vi "Fiducical Parameters Finder with joystick.vi"() -> ()   [LabVIEW 2011]
uses:
  Shared Components/Gantry Class/Type Definitions/Init_Modes.ctl
  Shared Components/Gantry Class/Gantry Class.lvclass
  Shared Components/Config Manager Class/Type Definitions/Camera Enum.ctl
  Shared Components/gVision API/gVision/gVision.lvlib
panel:
  out "error out":errorcluster
  in  "Find Fiducial":bool
  out "Preview":T1(plugin-control)
  in  "Stop":bool
  in  "Display Steps":bool
  out "Result":T1(plugin-control)
  out "ficucial coordinates":cluster{"x":dbl, "y":dbl}[](array[cluster])
  in  "Fiducial Parameters":T2
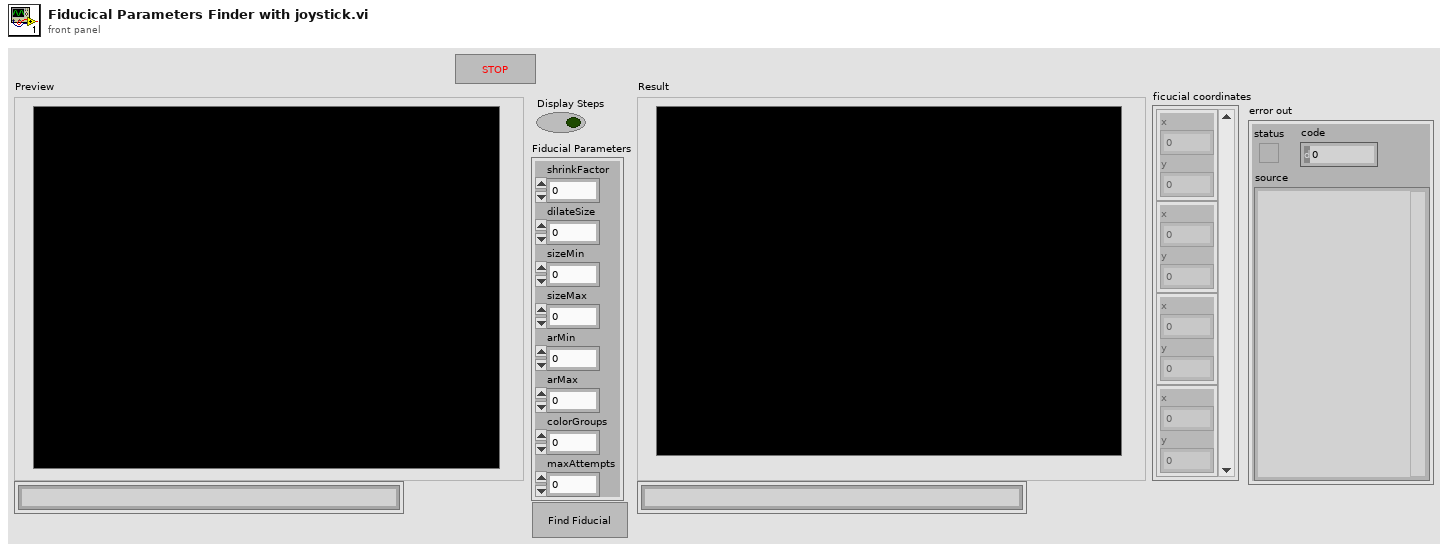
[diagram p1: front panel]
types:
  T1 = typedef "IMAQ Image.ctl" = refnum<image>
  T2 = cluster{"shrinkFactor":sgl, "dilateSize":i32, "sizeMin":sgl, "sizeMax":sgl, "arMin":sgl, "arMax":sgl, "colorGroups":i32, "maxAttempts":i32}
  T3 = typedef "Init_Modes.ctl" = enum16{"Full", "Robot Only", "Dispenser Only", "Cameras Only", "Robot and Cameras", "Robot and Cameras and Dispenser"}
  T4 = cluster{"Left":i32, "Top":i32, "Right":i32, "Bottom":i32}
  T5 = typedef "Camera Enum.ctl" = enum16{"GANTRY HEAD", "NEEDLE CALIBRATION X", "NEEDLE CALIBRATION Y", "STAND CAMERA"}
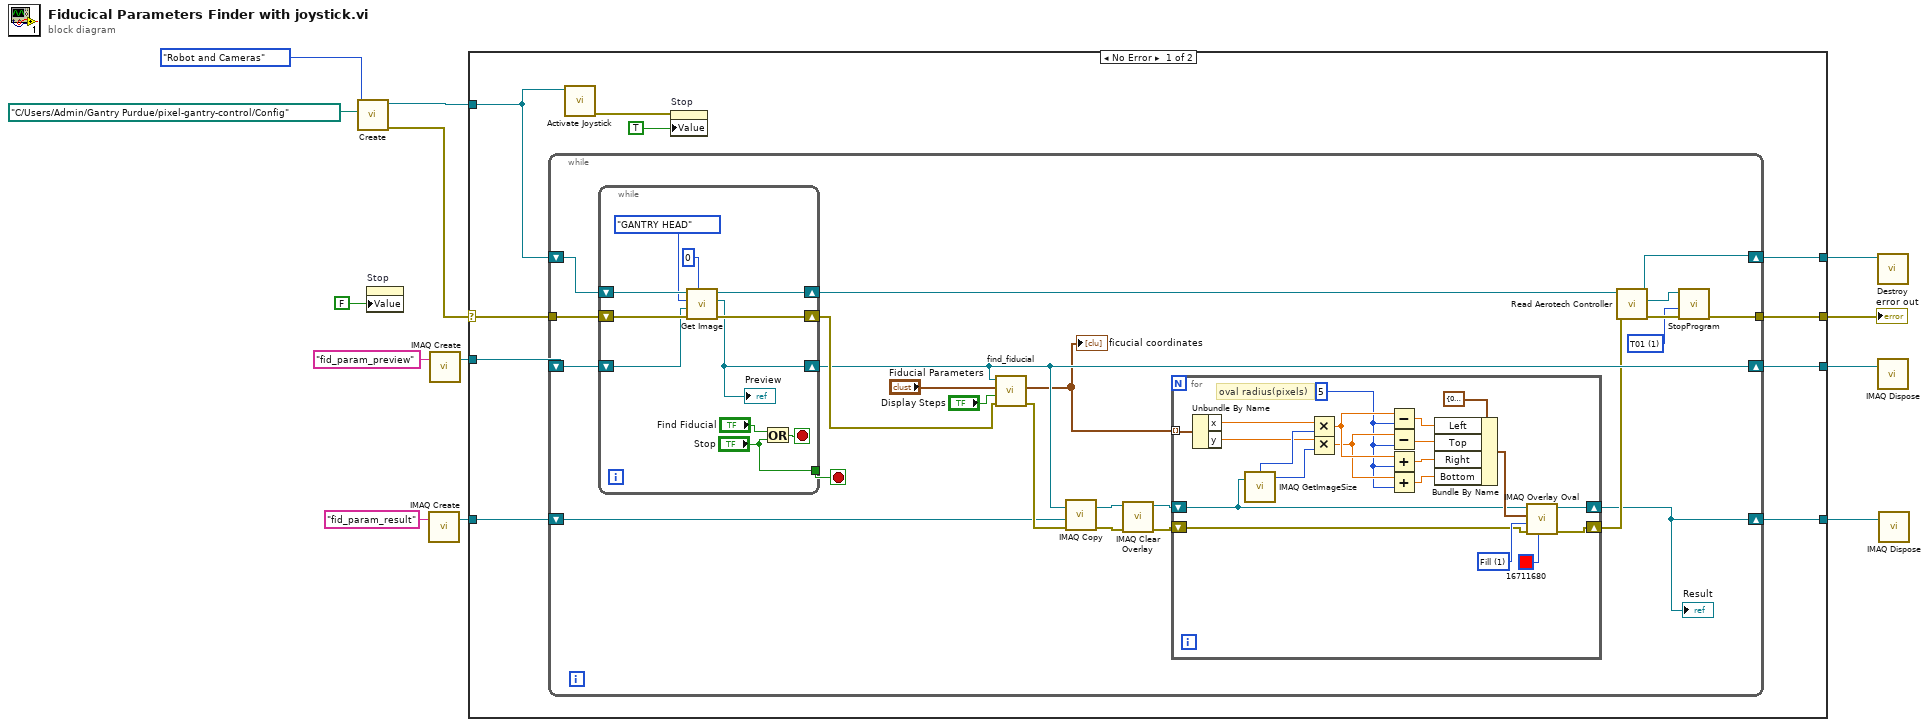
[diagram p0: block diagram]
diagram:
  n1 = call "Create.vi"("Config Folder"=path "C:/Users/Admin/Gantry Purdue/pixel-gantry-control/Config", "Init Mode"=Init_Modes."Robot and Cameras") -> ("error out"=w6:errorcluster, "Gantry out"=w7:refnum<class "Gantry Class.lvclass">)  [unwired: 8 in]
  n2 = property on="Stop" class="Bool (strict)"("Value"=FALSE ("Stop")) -> ()  [unwired: 2 in, 2 out]
  n3 = call "IMAQ Create"("Image Name"="fid_param_result") -> ("New Image"=w9:T1)  [unwired: 4 in, 1 out]
  n4 = call "IMAQ Create"("Image Name"="fid_param_preview") -> ("New Image"=w13:T1)  [unwired: 4 in, 1 out]
  n5 = case shown="No Error" w6 {
    selector: w6 -> [w20 w79]
    tunnel: w13 -> [w23 w81]
    tunnel: [w22 w81] -> w12
    tunnel: w9 -> [w15 w78]
    tunnel: w7 -> [w21 w80]
    tunnel: [w14 w79] -> w3
    tunnel: [w17 w80] -> w8
    tunnel: [w16 w78] -> w1
    frame No Error {
      n6 = while {
        tunnel: w20 -> [w46]
        shift-right: [w40] -> w22
        shift-left: w23 -> [w44]
        shift-right: [w28] -> w17
        shift-left: w21 -> [w45]
        tunnel: [w25] -> w14
        shift-right: [w24] -> w16
        shift-left: w15 -> [w27]
        stop <- w41 stop-if-true
        w31 = 1 items=["TLibrary", "T01", "T02", "T03", "T04", "T05", "T06", "T07", "T08", "T09", "T10", "T11", "T12", "T13", "T14", "T15", "T16", "T17", "T18", "T19", "T20", "T21", "T22", "T23", "T24", "T25", "T26", "T27", "T28", "T29", "T30", "T31"] ("taskId")
        n7 = while {
          shift-right: [w72] -> w40
          shift-left: w44 -> [w75]
          shift-right: [w74] -> w29
          shift-left: w45 -> [w76]
          shift-right: [w73] -> w42
          shift-left: w46 -> [w77]
          tunnel: ["Stop"] -> w41
          stop <- w70 stop-if-true
          n8 = call-dynamic "Get Image.vi"("Delay(milliseconds)"=0, "error in"=w77, "Image In"=w75, "Camera Name"=Camera_Enum."GANTRY HEAD", "Gantry in"=w76) -> ("error out"=w73:errorcluster, "Image Out"=w72:T1, "Gantry out"=w74:refnum<class "Gantry Class.lvclass">)  [unwired: 3 in, 1 out]
          "Preview" <- w72
          n9 = Or(x="Find Fiducial", y="Stop") -> (x .or. y?=w70:bool)
        }
        n10 = call "find_fiducial.vi"("error in"=w42, "interactive"="Display Steps", "Fiducial Parameters"="Fiducial Parameters", "Image"=w40) -> ("error out"=w38:errorcluster, "coords"=w39:cluster{"x":dbl, "y":dbl}[])  [unwired: 6 in]
        "ficucial coordinates" <- w39
        n11 = call "IMAQ Copy"("error in (no error)"=w38, "Image Dst"=w27, "Image Src"=w40) -> ("error out"=w36:errorcluster, "Image Dst Out"=w37:T1)  [unwired: 3 in]
        n12 = call "IMAQ Clear Overlay"("error in (no error)"=w36, "Image"=w37) -> ("error out"=w34:errorcluster, "Image Out"=w35:T1)  [unwired: 8 in]
        n13 = for {
          tunnel: w39 -> [w62] mode=indexing
          shift-right: [w66] -> w24
          shift-left: w35 -> [w58]
          shift-right: [w60] -> w26
          shift-left: w34 -> [w59]
          w47 = 5
          w61 = u32 1 items=["Frame", "Fill"] ("Drawing Mode (Frame)")
          # "oval radius(pixels)"
          n14 = Unbundle By Name(w62) -> ("x"=w56:dbl, "y"=w54:dbl)
          n15 = call "IMAQ GetImageSize"("Image"=w58) -> ("Y Resolution"=w55:i32, "X Resolution"=w57:i32)  [unwired: 3 in, 1 out]
          n16 = Multiply(x=w56, y=w57) -> (x*y=w49:dbl)
          n17 = Multiply(x=w54, y=w55) -> (x*y=w48:dbl)
          n18 = Subtract(x=w49, y=w47) -> (x-y=w53:dbl)
          n19 = Subtract(x=w48, y=w47) -> (x-y=w52:dbl)
          n20 = Add(x=w49, y=w47) -> (x+y=w51:dbl)
          n21 = Add(x=w48, y=w47) -> (x+y=w50:dbl)
          n22 = Bundle By Name(cluster=T4 {"Left"=0, "Top"=0, "Right"=0, "Bottom"=0} ("Bounding Rectangle"), "Left"=w53, "Top"=w52, "Right"=w51, "Bottom"=w50) -> (w63:T4)
          n23 = call "IMAQ Overlay Oval"("Color"=u32 16711680, "error in (no error)"=w59, "Drawing Mode (Frame)"=w61, "Bounding Rectangle"=w63, "Image"=w58) -> ("error out"=w60:errorcluster, "Image Out"=w66:T1)  [unwired: 5 in]
        }
        "Result" <- w24
        n24 = call-dynamic "Read Aerotech Controller.vi"("error in (no error)"=w26, "Gantry Class in"=w29) -> ("error out"=w32:errorcluster, "Aerotech Controller"=w30:refnum<k24>, "Gantry Class out"=w28:refnum<class "Gantry Class.lvclass">)  [unwired: 7 in]
        n25 = call <userlib>:"StopProgram.vi"("error in (no error)"=w32, "taskId"=w31, "controller in"=w30) -> ("error out"=w25:errorcluster)  [unwired: 7 in, 1 out]
      }
      n26 = call-dynamic "Activate Joystick.vi"("Gantry Class in"=w21) -> ("error out"=w18:errorcluster)  [unwired: 9 in, 1 out]
      n27 = property on="Stop" class="Bool (strict)"(error in=w18, "Value"=TRUE ("stop")) -> ()  [unwired: 1 in, 2 out]
    }
    frame Error {
    }
  }
  "error out" <- w3
  n28 = call "Destroy.vi"("Gantry Class in"=w8) -> ()  [unwired: 10 in, 1 out]
  n29 = call "IMAQ Dispose"("Image"=w12) -> ()  [unwired: 5 in, 1 out]
  n30 = call "IMAQ Dispose"("Image"=w1) -> ()  [unwired: 5 in, 1 out]
